vi "Read AppOutput.vi"(8 "error in (no error)":errorcluster, 11 "VisualizeAppRingdown in":refnum<class "VisualizeAppERA.lvclass">) -> (0 "error out":errorcluster, 2 "RingdownOutput":T1, 3 "VisualizeAppRingdown out":refnum<class "VisualizeAppERA.lvclass">)   [LabVIEW 2017, in "Visualization.lvlib" / "VisualizeAppERA.lvclass"]
uses:
  VisualizeAppERA.lvclass
  Modules/AppPlugins/EraPlugin/PublicAPI/TypeDef/ERAOutput.ctl
  VisualizeAppERA.lvclass/VisualizeAppERA.ctl
  Modules/AppPlugins/EraPlugin/EraPlugin.lvclass
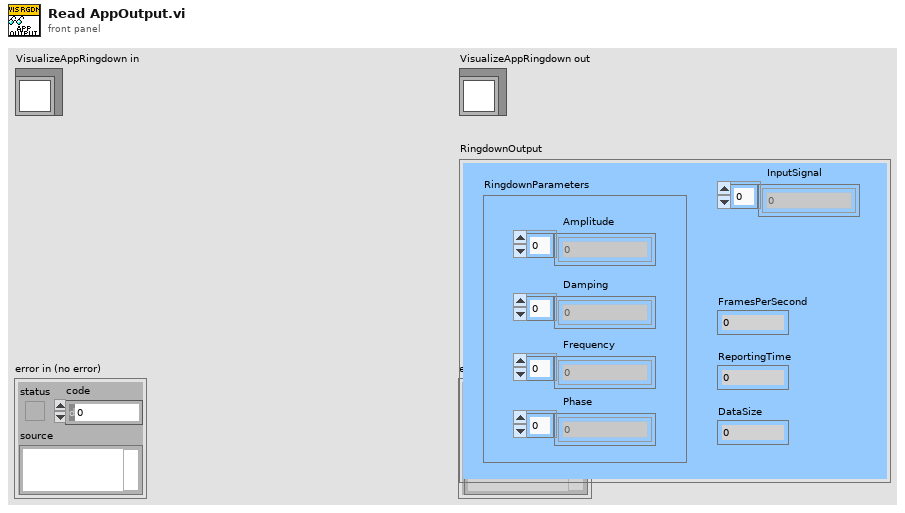
[diagram p1: front panel]
types:
  T1 = typedef "AppPlugins.lvlib/ERAPlugin.lvclass/ERAOutput.ctl" = cluster{"FramesPerSecond":dbl, "RingdownParameters":cluster{"Amplitude":dbl[], "Damping":dbl[], "Frequency":dbl[], "Phase":dbl[]}, "ReportingTime":dbl, "DataSize":u32, "InputSignal":dbl[]}
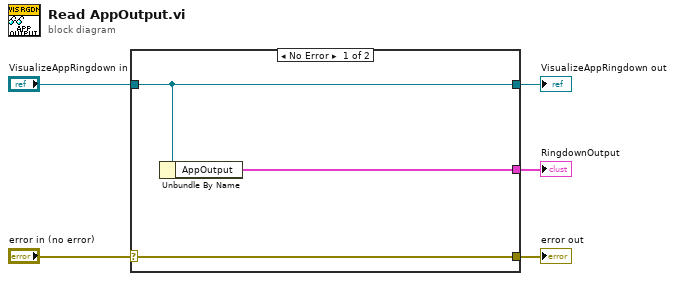
[diagram p0: block diagram]
diagram:
  n1 = case shown="No Error" "error in (no error)" {
    selector: "error in (no error)" -> [w8 w9]
    tunnel: [w8 w9] -> w4
    tunnel: [w7 w10] -> w2
    tunnel: "VisualizeAppRingdown in" -> [w7 w10]
    tunnel: [w6 _] -> w1
    frame No Error {
      n2 = Unbundle By Name(w7) -> ("AppOutput"=w6:T1)
    }
    frame Error {
    }
  }
  "error out" <- w4
  "VisualizeAppRingdown out" <- w2
  "RingdownOutput" <- w1
